vi "Simulate Video Hardware.vi"(7 "Command to Simulate":T2=enum."Simulate Read HDMI Data", 8 "error in (no error)":errorcluster, 10 "Simulation Data":T1={"PowerOn"=TRUE, "Battery"=TRUE, "Antenna"=TRUE, "Microphone"=TRUE, "Speakers"=TRUE, "Buttons"=TRUE, "LCD"=enum."Passing Image"}, 11 "Test Image Data":u32[][](array[numeric])) -> (0 "error out":errorcluster, 3 "UUT Image Data Out":u32[][](array[numeric]))   [LabVIEW 2011]
uses:
  Video Hardware Simulation Commands.ctl
  Simulation Data.ctl
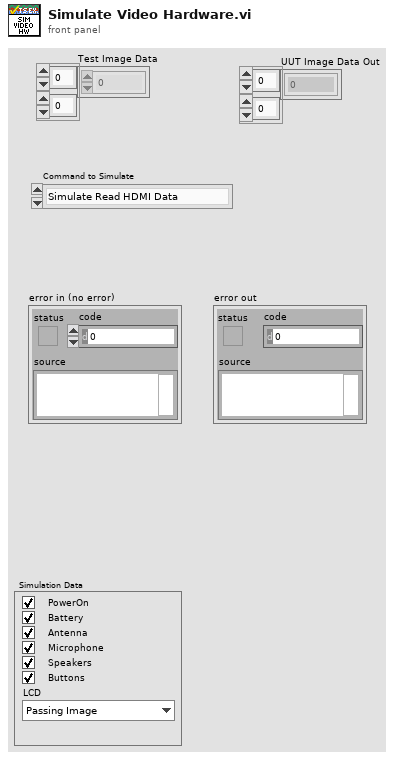
[diagram p1: front panel]
types:
  T1 = typedef "Simulation Data.ctl" = cluster{"PowerOn":bool, "Battery":bool, "Antenna":bool, "Microphone":bool, "Speakers":bool, "Buttons":bool, "LCD":enum16{"Passing Image", "Dead Pixels", "Incorrect Brightness"}}
  T2 = typedef "Video Hardware Simulation Commands.ctl" = enum16{"Simulate Generate Video Output", "Simulate Read HDMI Data"}
  T3 = enum16{"Passing Image", "Dead Pixels", "Incorrect Brightness"}
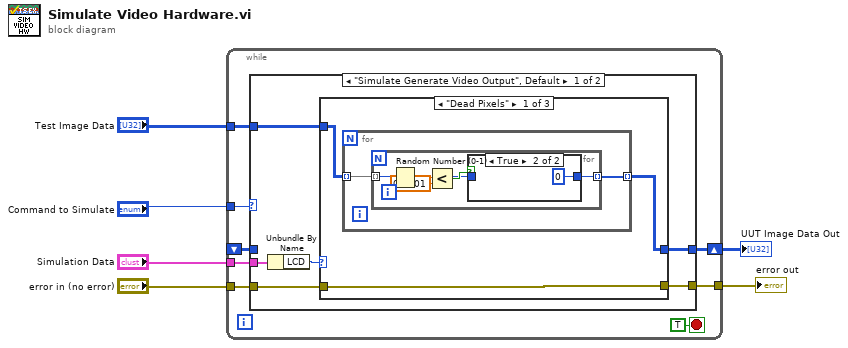
[diagram p0: block diagram]
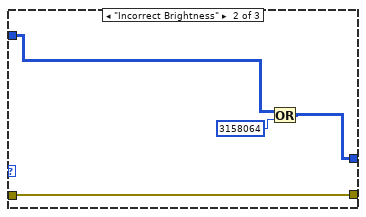
[diagram p3: hidden frame]
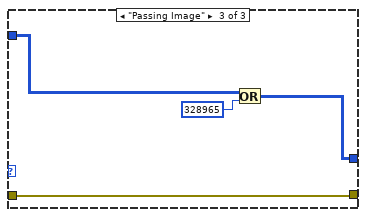
[diagram p4: hidden frame]
diagram:
  n1 = while {
    tunnel: [w13] -> w6
    tunnel: "error in (no error)" -> [w12]
    tunnel: "Command to Simulate" -> [w11]
    shift-right: [w14] -> w2
    shift-left: _ -> [w10]
    tunnel: "Test Image Data" -> [w8]
    tunnel: "Simulation Data" -> [w7]
    stop <- TRUE stop-if-true
    n2 = case shown="\"Simulate Generate Video Output\", Default" w11 {
      tunnel: [w20 w42] -> w14
      tunnel: [w18 w41] -> w13
      tunnel: w12 -> [w19 w41]
      tunnel: w10 -> [_ w42]
      tunnel: w8 -> [w15 _]
      tunnel: w7 -> [w17 _]
      frame "Simulate Generate Video Output", Default {
        n3 = Unbundle By Name(w17) -> ("LCD"=w16:T3)
        n4 = case shown="\"Dead Pixels\"" w16 {
          tunnel: [w22 w34 w39] -> w20
          tunnel: w19 -> [w21 w36 w38]
          tunnel: [w21 w36 w38] -> w18
          tunnel: w15 -> [w23 w33 w40]
          frame "Dead Pixels" {
            n5 = for {
              tunnel: w23 -> [w25] mode=indexing
              tunnel: [w24] -> w22 mode=indexing
              n6 = for {
                tunnel: w25 -> [w27] mode=indexing
                tunnel: [w26] -> w24 mode=indexing
                n7 = Random Number (0-1)() -> (number: 0 to 1=w30:dbl)
                n8 = Less?(x=w30, y=0.0001) -> (x < y?=w28:bool)
                n9 = case shown="True" w28 {
                  tunnel: w27 -> [w31 _]
                  tunnel: [w31 u32 0] -> w26
                  frame False {
                  }
                  frame True {
                  }
                }
              }
            }
          }
          frame "Incorrect Brightness" {
            n10 = Or(x=w33, y=u32 3158064) -> (x .or. y?=w34:u32[][])
          }
          frame "Passing Image" {
            n11 = Or(x=w40, y=u32 328965) -> (x .or. y?=w39:u32[][])
          }
        }
      }
      frame "Simulate Read HDMI Data" {
      }
    }
  }
  "error out" <- w6
  "UUT Image Data Out" <- w2
